vi "Get Packet Data.vi"(0 "Network Actor in":refnum<class "Network Actor.lvclass">) -> ()   [LabVIEW 2018, in "Network Actor Library.lvlib" / "Network Actor.lvclass"]
uses:
  Network Actor.lvclass
  C:/Users/Labview/Documents/exscalabar_server/SuperActor/SuperActor.lvclass
  Network Actor.lvclass/Network Actor.ctl
  SuperActor/SuperActor.lvclass/SuperActor.ctl
  SuperActor/Read Log Session.vi
  <userlib>/_Session Fwk/Session - Root.lvclass
  reusable/Session APIs/Session Log/System Log.lvclass
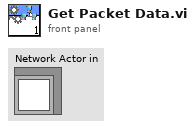
[diagram p1: front panel]
types:
  T1 = cluster{"ID":string, "DataDescr":cluster{"Type":string, "Name":string, "Write":bool}[]}[]
  T2 = typedef "Session - Root.lvclass/Session Handle.ctl" = refnum<data-value>
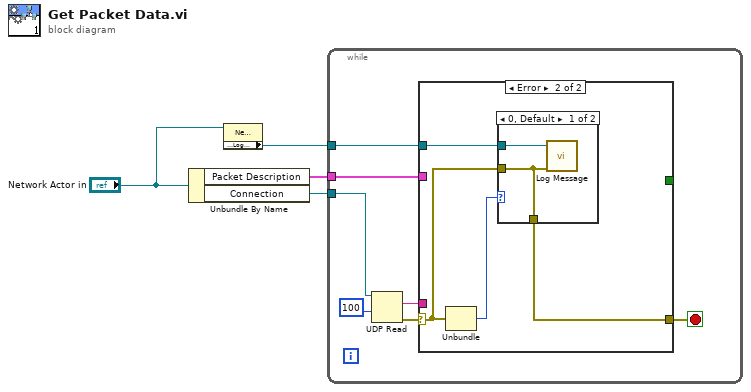
[diagram p0: block diagram]
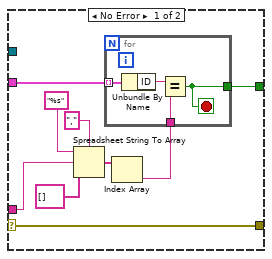
[diagram p2: hidden frame]
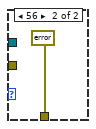
[diagram p3: hidden frame]
diagram:
  n1 = Unbundle By Name("Network Actor in") -> ("Packet Description"=w3:T1, "Connection"=w4:refnum<k16>)
  n2 = property class="Network Actor"(reference="Network Actor in") -> ("Accessors:Log Session"=w1:T2)  [unwired: 1 in, 2 out]
  n3 = while {
    tunnel: w4 -> [w10]
    tunnel: w3 -> [w6]
    tunnel: w1 -> [w5]
    stop <- w8 stop-if-true
    n4 = UDP Read(connection ID=w10, timeout ms (25000)=100) -> (data out=w7:string, error out=w9:errorcluster)  [unwired: 1 in, 4 out]
    n5 = case shown="Error" w9 {
      selector: w9 -> [w20 w26]
      tunnel: w5 -> [_ w28]
      tunnel: [w20 w25] -> w8
      tunnel: w7 -> [w19 _]
      tunnel: w6 -> [w15 _]
      tunnel: [w12 _] -> _
      frame No Error {
        n6 = Spreadsheet String To Array(delimiter (Tab)=",", format string="%s", spreadsheet string=w19, array type (2D Dbl)=string[] []) -> (array=w14:string[])
        n7 = Index Array(array=w14) -> (element=w13:string)  [unwired: 1 in]
        n8 = for {
          tunnel: w15 -> [w24] mode=indexing
          tunnel: w13 -> [w22]
          tunnel: [w21] -> w12
          stop <- w21 stop-if-true
          n9 = Unbundle By Name(w24) -> ("ID"=w23:string)
          n10 = Equal?(x=w23, y=w22) -> (x = y?=w21:bool)
        }
      }
      frame Error {
        n11 = Unbundle(w26) -> ("code"=w27:i32)  [unwired: 2 out]
        n12 = case shown="0, Default" w27 {
          tunnel: w28 -> [w30 _]
          tunnel: w26 -> [w29 _]
          tunnel: [w29 errorcluster {"status"=FALSE, "code"=0, "source"=""} ("error IO")] -> w25
          frame 0, Default {
            n13 = call "Log Message.vi"("error in"=w29, "session in"=w30) -> ()  [unwired: 8 in, 2 out]
          }
          frame 56 {
          }
        }
      }
    }
  }
